vi "test_libssh2_channel_window_read_ex.vi"() -> ()   [LabVIEW 2017, in "integration_tests.lvlib"]
uses:
  integration_tests.lvlib
  libssh2/libssh2_channel_open_ex.vi
  support/support.lvlib
  libssh2/libssh2.lvlib
  <vilib>/PNR/Transparent Assertions/Transparent Assertions/Transparent Assertions.lvlib
panel:
  out "error out":errorcluster
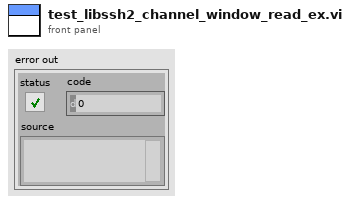
[diagram p1: front panel]
types:
  T1 = typedef "libssh2.lvlib/Session Refnum.ctl" = refnum<k1>
  T2 = typedef "libssh2.lvlib/Channel Refnum.ctl" = refnum<k1>
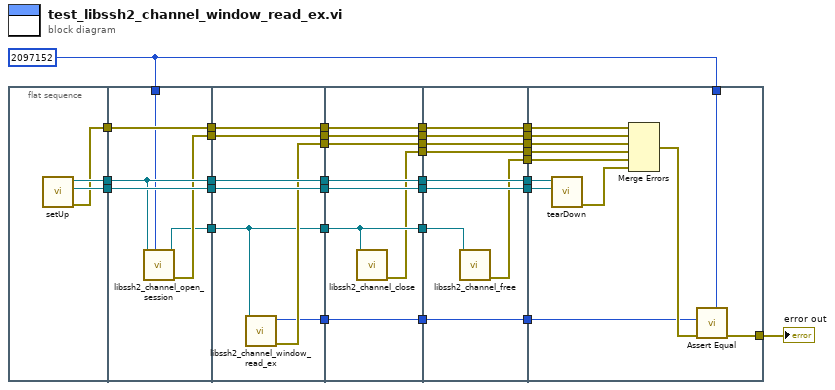
[diagram p0: block diagram]
diagram:
  w2 = u32 2097152 ("window_size (2 MiB)")
  n1 = flat-sequence {
    tunnel: [w36] -> w33
    tunnel: [w35] -> w32
    tunnel: [w34] -> w31
    tunnel: w33 -> [w41]
    tunnel: w32 -> [w42]
    tunnel: [w41] -> w7
    tunnel: [w42] -> w6
    tunnel: w31 -> [w40]
    tunnel: [w40] -> w5
    tunnel: [w39] -> w4
    tunnel: w2 -> [w38]
    tunnel: [w37] -> w3
    tunnel: w7 -> [w49]
    tunnel: [w49] -> w30
    tunnel: w6 -> [w48]
    tunnel: [w48] -> w29
    tunnel: [w43] -> w28
    tunnel: w5 -> [w47]
    tunnel: [w47] -> w27
    tunnel: w4 -> [w46]
    tunnel: [w46] -> w26
    tunnel: [w45] -> w25
    tunnel: [w44] -> w24
    tunnel: w3 -> [w43]
    tunnel: w30 -> [w57]
    tunnel: w29 -> [w56]
    tunnel: w28 -> [w55]
    tunnel: [w57] -> w23
    tunnel: [w56] -> w22
    tunnel: [w50] -> w21
    tunnel: [w55] -> w20
    tunnel: [w54] -> w19
    tunnel: w27 -> [w53]
    tunnel: [w53] -> w18
    tunnel: w26 -> [w52]
    tunnel: [w52] -> w17
    tunnel: w25 -> [w51]
    tunnel: [w51] -> w16
    tunnel: w24 -> [w50]
    tunnel: w23 -> [w66]
    tunnel: w22 -> [w65]
    tunnel: w21 -> [w64]
    tunnel: w20 -> [w63]
    tunnel: [w66] -> w15
    tunnel: [w65] -> w14
    tunnel: [w64] -> w13
    tunnel: [w62] -> w12
    tunnel: w19 -> [w61]
    tunnel: [w61] -> w11
    tunnel: w18 -> [w60]
    tunnel: [w60] -> w10
    tunnel: w17 -> [w59]
    tunnel: [w59] -> w9
    tunnel: w16 -> [w58]
    tunnel: [w58] -> w8
    tunnel: w15 -> [w78]
    tunnel: w14 -> [w77]
    tunnel: w13 -> [w68]
    tunnel: [w76] -> w1
    tunnel: w12 -> [w74]
    tunnel: w11 -> [w73]
    tunnel: w10 -> [w72]
    tunnel: w9 -> [w70]
    tunnel: w8 -> [w69]
    tunnel: w2 -> [w67]
    frame #0 {
      n2 = call "setUp.vi"() -> ("error out"=w34:errorcluster, "connection ID"=w35:refnum<k5>, "session"=w36:T1)  [unwired: 9 in]
    }
    frame #1 {
      n3 = call "libssh2_channel_open_session.vi"("window_size (2 MiB)"=w38, "session"=w41) -> ("error out"=w39:errorcluster, "channel"=w37:T2)  [unwired: 8 in]
    }
    frame #2 {
      n4 = call "libssh2_channel_window_read_ex.vi"("channel"=w43) -> ("error out"=w45:errorcluster, "remaining read window"=w44:u32)  [unwired: 7 in, 2 out]
    }
    frame #3 {
      n5 = call "libssh2_channel_close.vi"("channel"=w55) -> ("error out"=w54:errorcluster)  [unwired: 10 in]
    }
    frame #4 {
      n6 = call "libssh2_channel_free.vi"("channel"=w63) -> ("error out"=w62:errorcluster)  [unwired: 10 in]
    }
    frame #5 {
      n7 = call "tearDown.vi"("connection ID"=w77, "session"=w78) -> ("error out"=w75:errorcluster)  [unwired: 9 in]
      n8 = Merge Errors(w72, w70, w69, w73, w74, w75) -> (w71:errorcluster)
      n9 = call <vilib>:"Assert Equal.vi"("Expected"=w67, "error in (no error)"=w71, "Actual"=w68) -> ("error out"=w76:errorcluster)  [unwired: 8 in]
    }
  }
  "error out" <- w1
